vi "从数据库同步累积剂量.vi"(6 "error in (no error)":errorcluster, 7 "累积剂量 i":T2(array[cluster]) caption="累积剂量", 11 "数据库连接引用 i":T1) -> (1 "表名":string[](array[string]), 3 "数据库连接引用 o":T1, 4 "error out":errorcluster, 5 "累积剂量 o":T2(array[cluster]) caption="累积剂量")   [LabVIEW 2017]
uses:
  <vilib>/addons/database/Connection.llb/Conn ObjectReference.ctl
  <vilib>/addons/database/NI_Database_API.lvlib
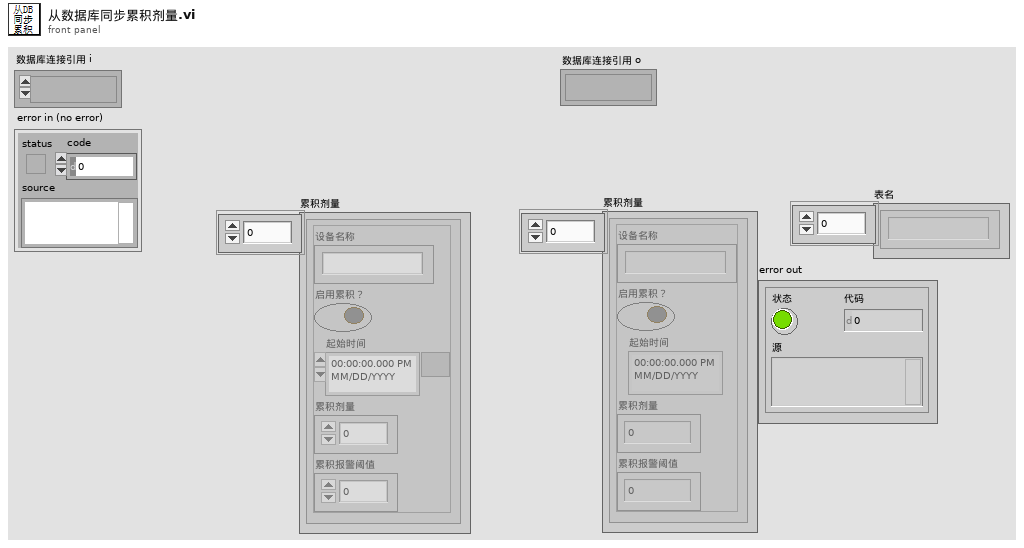
[diagram p1: front panel]
types:
  T1 = typedef "NI_Database_API.lvlib/Conn ObjectReference.ctl" = refnum<k1>
  T2 = cluster{"设备名称":string, "启用累积？":bool, "起始时间":timestamp, "累积剂量":dbl, "累积报警阈值":dbl}[]
  T3 = cluster{"设备名称":string, "启用累积？":bool, "起始时间":timestamp, "累积剂量":dbl, "累积报警阈值":dbl}
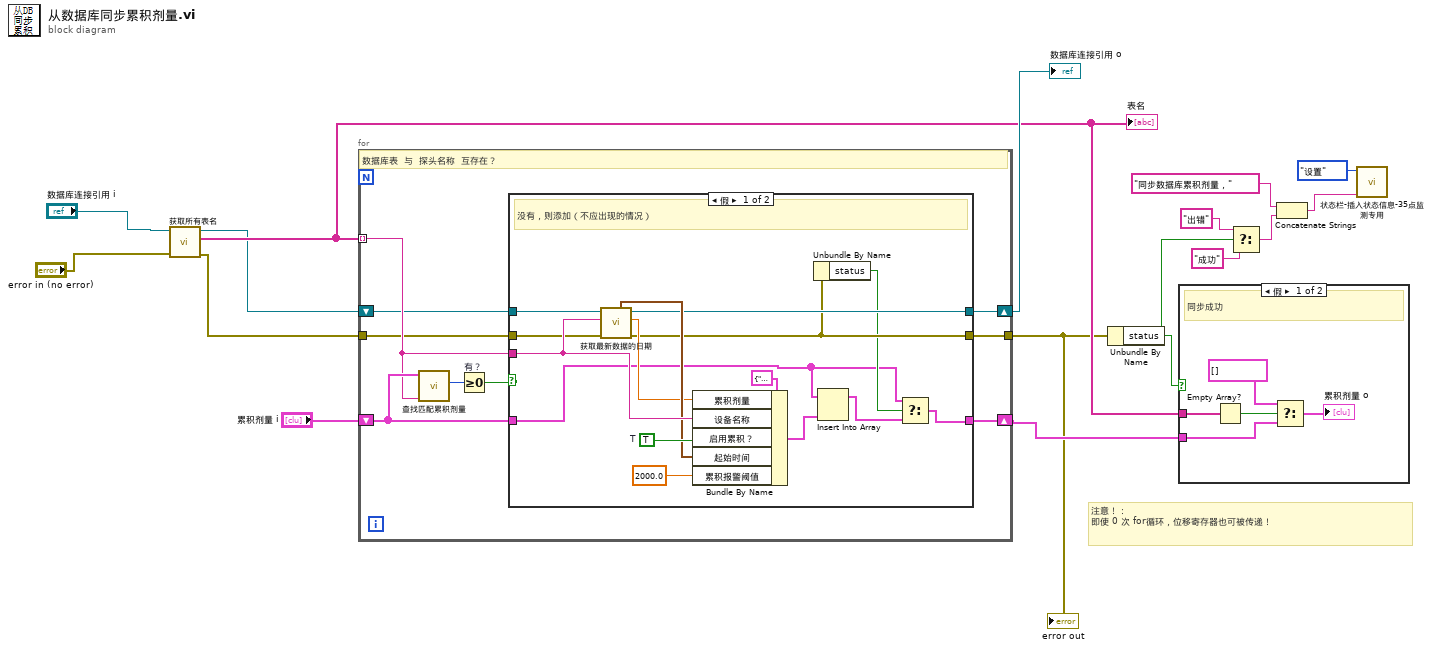
[diagram p0: block diagram]
diagram:
  # "注意！：\n即使 0 次 for循环，位移寄存器也可被传递！"
  n1 = call "获取所有表名.vi"("error in (no error)"="error in (no error)", "数据库连接引用 i"="数据库连接引用 i") -> ("error out"=w6:errorcluster, "表名"=w13:string[], "数据库连接引用 o"=w5:T1)  [unwired: 7 in]
  "表名" <- w13
  n2 = for {
    tunnel: w13 -> [w23] mode=indexing
    shift-right: [w25] -> w14
    shift-left: "累积剂量 i" -> [w24]
    tunnel: w6 -> [w19]
    tunnel: [w18] -> w12
    shift-right: [w17] -> w16
    shift-left: w5 -> [w20]
    # "数据库表  与  探头名称  互存在？"
    n3 = call "查找匹配累积剂量.vi"("探头名称"=w23, "累积剂量"=w24) -> ("匹配索引"=w21:i32)  [unwired: 7 in, 2 out]
    n4 = Greater Or Equal To 0? "有？"(x=w21) -> (x >= 0?=w22:bool)
    n5 = case shown="假" w22 {
      tunnel: w24 -> [w28 w43]
      tunnel: [w26 w43] -> w25
      tunnel: w23 -> [w35 _]
      tunnel: w20 -> [w36 w42]
      tunnel: w19 -> [w34 w41]
      tunnel: [w31 w42] -> w17
      tunnel: [w30 w41] -> w18
      frame False {
        w39 = TRUE  # T
        # "没有，则添加（不应出现的情况）"
        n6 = call "获取最新数据的日期.vi"("error in (no error)"=w34, "表名"=w35, "数据库连接引用 i"=w36) -> ("error out"=w30:errorcluster, "累积值"=w32:dbl, "数据库连接引用 o"=w31:T1, "起始时间"=w33:timestamp)  [unwired: 4 in, 1 out]
        n7 = Bundle By Name(cluster=T3 {"设备名称"="", "启用累积？"=TRUE, "起始时间"=timestamp(0 s since 1904-01-01), "累积剂量"=0.0, "累积报警阈值"=2000.0} ("新元素/子数组"), "累积剂量"=w32, "设备名称"=w35, "启用累积？"=w39, "起始时间"=w33, "累积报警阈值"=2000.0) -> (w37:T3)
        n8 = Unbundle By Name(w30) -> ("status"=w29:bool)
        n9 = Insert Into Array(array=w28, new element=w37) -> (w27:T2)  [unwired: 1 in]
        n10 = Select(t=w28, s=w29, f=w27) -> (s? t:f=w26:T2)
      }
      frame True {
        # "有，则通过"
      }
    }
  }
  "数据库连接引用 o" <- w16
  "error out" <- w12
  n11 = Unbundle By Name(w12) -> ("status"=w15:bool)
  n12 = case shown="假" w15 {
    tunnel: w13 -> [w48 _]
    tunnel: w14 -> [w45 _]
    frame False {
      # "同步成功"
      n13 = Empty Array?(array=w48) -> (empty?=w47:bool)
      n14 = Select(t=T2 [] ("累积剂量"), s=w47, f=w45) -> (s? t:f=→"累积剂量 o":T2)
    }
    frame True {
      # "同步错误，不修改变量"
    }
  }
  n15 = Select(t="出错" ("消息内容"), s=w15, f="成功" ("消息内容")) -> (s? t:f=w10:string)
  n16 = Concatenate Strings("同步数据库累积剂量，" ("消息内容"), w10) -> (w11:string)
  n17 = call "状态栏-插入状态信息-35点监测专用.vi"("消息内容"=w11, "状态类型"=enum16{"全部", "报警", "通信", "设置"}."设置") -> ()  [unwired: 10 in]
